vi "Ev Reset Path.vi"(8 "error in (no error)":errorcluster, 11 "Configuration Window in":refnum<class "Configuration Window.lvclass">) -> (0 "error out":errorcluster, 3 "Configuration Window out":refnum<class "Configuration Window.lvclass">)   [LabVIEW 2018, in "Configuration Window.lvlib" / "Configuration Window.lvclass"]
uses:
  Configuration Window.lvclass
  Configuration Window.lvclass/Configuration Window.ctl
  Main Panel/LF2R IDE/Main Panel.lvclass
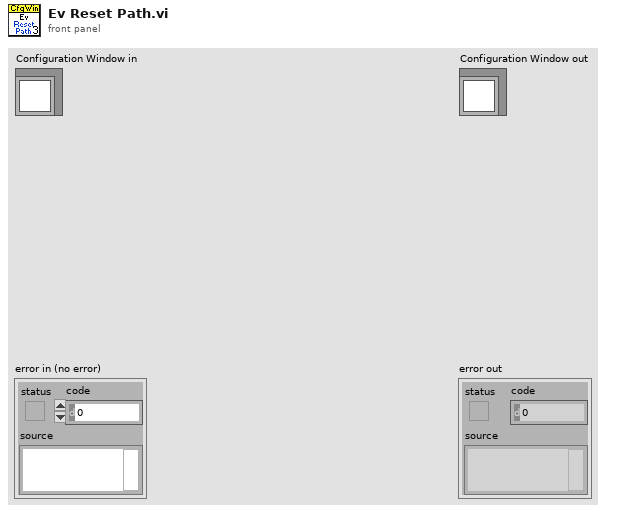
[diagram p1: front panel]
types:
  T1 = cluster{"LF2R Path":path, "Data Path":path, "PNG Path":path, "mp3 Path":path}
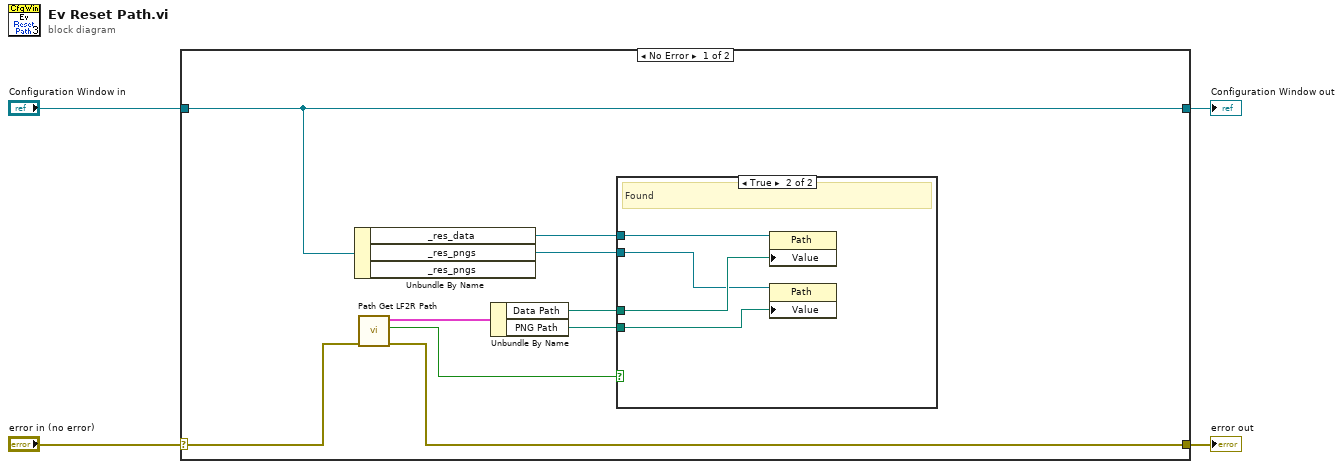
[diagram p0: block diagram]
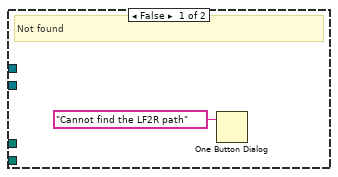
[diagram p2: hidden frame]
diagram:
  n1 = case shown="No Error" "error in (no error)" {
    selector: "error in (no error)" -> [w9 w20]
    tunnel: [w10 w20] -> w3
    tunnel: [w13 w19] -> w1
    tunnel: "Configuration Window in" -> [w13 w19]
    frame No Error {
      n2 = Unbundle By Name(w13) -> ("_res_data"=w12:refnum<vi>, "_res_pngs"=w11:refnum<vi>)  [unwired: 1 out]
      n3 = call "Path Get LF2R Path.vi"("error in (no error)"=w9) -> ("error out"=w10:errorcluster, "Found"=w8:bool, "Path"=w7:T1)  [unwired: 8 in]
      n4 = Unbundle By Name(w7) -> ("Data Path"=w6:path, "PNG Path"=w5:path)
      n5 = case shown="True" w8 {
        tunnel: w12 -> [_ w18]
        tunnel: w6 -> [_ w17]
        tunnel: w11 -> [_ w16]
        tunnel: w5 -> [_ w15]
        frame False {
          # "Not found"
          n6 = One Button Dialog(message="Cannot find the LF2R path") -> ()  [unwired: 1 in, 1 out]
        }
        frame True {
          # "Found"
          n7 = property class="Path"(reference=w18, "Value"=w17) -> ()  [unwired: 1 in, 2 out]
          n8 = property class="Path"(reference=w16, "Value"=w15) -> ()  [unwired: 1 in, 2 out]
        }
      }
    }
    frame Error {
    }
  }
  "error out" <- w3
  "Configuration Window out" <- w1
